vi "comments.vi"   [LabVIEW 2012]
uses:
  <vilib>/addons/internet/NI_InternetTK_Common_VIs.lvlib
  <vilib>/addons/internet/NI_InternetTK_Core_VIs.lvlib
types:
  T1 = typedef "CGI Connection Info.ctl" = cluster{"name":string, "type":T2, "session":T3}
  T2 = typedef "CGI Request Type.ctl" = enum16{"cgi", ".spool first", ".spool", ".spool last"}
  T3 = typedef "HTTP Session.ctl" = refnum<k1>
  T4 = typedef "NI_FTP.lvlib/Keyed Array.ctl" = cluster{"keys":string[], "values":string[]}
  T5 = typedef "comment.ctl" = cluster{"Time":dbl, "Name":string, "Comment":string}
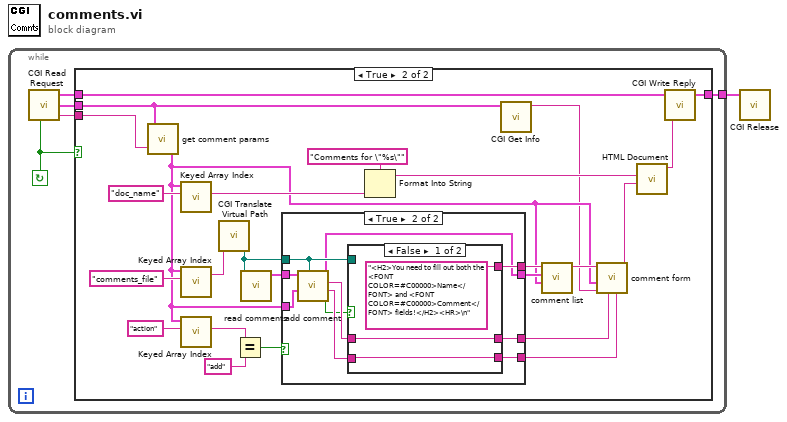
[diagram p0: block diagram]
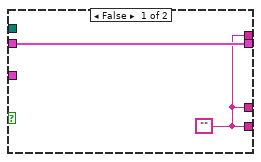
[diagram p3: hidden frame]
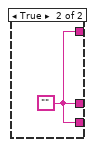
[diagram p4: hidden frame]
diagram:
  n1 = while {
    tunnel: [w6] -> w1
    stop <- w2 continue-if-true
    n2 = call <vilib>:"CGI Read Request.vi"() -> ("valid request?"=w2:bool, "cgi connection info"=w5:T1, "env"=w3:T4, "content"=w4:string)  [unwired: 4 in]
    n3 = case shown="True" w2 {
      tunnel: [w7 w31] -> w6
      tunnel: w5 -> [w7 w30]
      tunnel: w4 -> [_ w29]
      tunnel: w3 -> [_ w9]
      frame False {
      }
      frame True {
        n4 = call "get comment params.vi"("content"=w29, "env"=w9) -> ("params"=w10:T4)
        n5 = call <vilib>:"Keyed Array Index.vi"("key"="doc_name" ("name"), "array in"=w10) -> ("value"=w15:string)  [unwired: 3 in, 2 out]
        n6 = call <vilib>:"Keyed Array Index.vi"("key"="comments_file" ("name"), "array in"=w10) -> ("value"=w27:string)  [unwired: 3 in, 2 out]
        n7 = call <vilib>:"Keyed Array Index.vi"("key"="action" ("name"), "array in"=w10) -> ("value"=w17:string)  [unwired: 3 in, 2 out]
        n8 = call <vilib>:"CGI Translate Virtual Path.vi"("virtual path"=w27) -> ("absolute path"=w28:path)  [unwired: 1 in]
        n9 = Equal?(x=w17, y="add") -> (x = y?=w19:bool)
        n10 = call "read comments.vi"("file name"=w28) -> ("Comments"=w22:T5[])  [unwired: 10 in]
        n11 = case shown="True" w19 {
          tunnel: w22 -> [w34 w40]
          tunnel: [w34 w39] -> w23
          tunnel: w10 -> [_ w38]
          tunnel: w28 -> [_ w41]
          tunnel: [w33 w44] -> w24
          tunnel: [w33 w43] -> w25
          tunnel: [w33 w42] -> w26
          frame False {
            w33 = ""
          }
          frame True {
            n12 = call "add comment.vi"("comments file"=w41, "params"=w38, "comments in"=w40) -> ("valid"=w35:bool, "comment"=w36:string, "name"=w37:string, "comments out"=w39:T5[])  [unwired: 5 in]
            n13 = case shown="False" w35 {
              tunnel: w36 -> [w46 _]
              tunnel: w37 -> [w47 _]
              tunnel: w41 -> [_ _]
              tunnel: [w47 w48] -> w44
              tunnel: [w46 w48] -> w43
              tunnel: ["<H2>You need to fill out both the <FONT COLOR=#C00000>Name</FONT> and <FONT COLOR=#C00000>Comment</FONT> fields!</H2><HR>\n" w48] -> w42
              frame False {
              }
              frame True {
                w48 = ""
              }
            }
          }
        }
        n14 = Format Into String(format string="Comments for \"%s\"", w15) -> (resulting string=w14:string)  [unwired: 2 in, 1 out]
        n15 = call <vilib>:"CGI Get Info.vi"("env"=w9) -> ("cgi name"=w8:string)  [unwired: 4 in, 2 out]
        n16 = call "comment list.vi"("params"=w10, "Comments"=w23, "HTML In"=w26) -> ("HTML In Out"=w20:string)  [unwired: 8 in]
        n17 = call "comment form.vi"("Default Comment (\"\")"=w25, "Default Name (\"\")"=w24, "self"=w8, "params"=w10, "HTML In"=w20) -> ("HTML In Out"=w11:string)  [unwired: 6 in]
        n18 = call <vilib>:"HTML Document.vi"("document body"=w11, "document title"=w14) -> ("HTML Document"=w32:string)  [unwired: 9 in]
        n19 = call <vilib>:"CGI Write Reply.vi"("content"=w32, "cgi connection info"=w30) -> ("cgi connection info out"=w31:T1)  [unwired: 3 in]
      }
    }
  }
  n20 = call <vilib>:"CGI Release.vi"("cgi connection info"=w1) -> ()  [unwired: 5 in]
